vi "Pascal Case to Standard.vi"(8 "error in (no error)":errorcluster, 11 "Input String":string) -> (0 "error out":errorcluster, 3 "Output String":string)   [LabVIEW 2015, in "Case Manipulation.lvlib"]
doc: "Introduction:\nWe often remove the spaces between words because programs of different sorts reserve the space (‘ ’) character for special purposes. Because the space character is reserved, we cannot use it to represent a concept that we express in our human language with multiple words.\nPascal Case:\nThis is also a very popular way to combine words to form a single concept. It is often used as a convention in declaring classes in many languages."
uses:
  Case Manipulation.lvlib
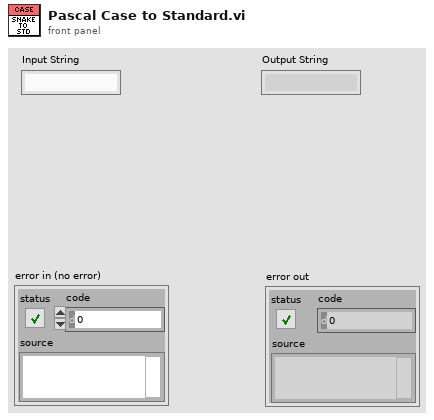
[diagram p1: front panel]
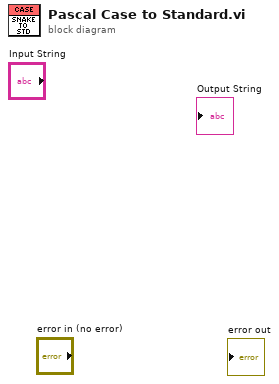
[diagram p0: block diagram]
diagram:
